vi "Set time.vi"(6 "Defer restart? (true)":bool=TRUE, 8 "error in (no error)":errorcluster, 10 "Time zone":T1 items=["UTC/GMT"=0, "[GMT-1]Azores, Cape Verde"=1, "[GMT-2] Falkland Islands"=2, "[GMT-3] Greenland, East Brazil"=3, "[GMT-4] Central Brazil"=4, "[GMT-5] Eastern United States, Colombia"=5, "[GMT-6] Central United States, Honduras"=6, "[GMT-7] Mountain United States"=7, "[GMT-8] Pacific United States, Yukon"=8, "[GMT-9] Alaska"=9, "[GMT-10] Hawaii, Aleutian Islands"=10, "[GMT-11] Bering Strait"=11, "[GMT+12] New Zealand"=-12, "[GMT+11] Solomon Islands"=-11, "[GMT+10] Eastern Australia"=-10, "[GMT+9] Japan/Korea"=-9, "[GMT+8] Western Australia, Taiwan"=-8, "[GMT+7] Thailand"=-7, "[GMT+6] Central Asia"=-6, "[GMT+5] Pakistan"=-5, "[GMT+4] Gorki, Central Asia, Oman"=-4, "[GMT+3] Turkey, Saudi Arabia"=-3, "[GMT+2] Finland, South Africa"=-2, "[GMT+1] Norway"=-1], 11 "RT Management in":refnum<class "RT Management.lvclass">) -> (0 "error out":errorcluster, 3 "RT Management out":refnum<class "RT Management.lvclass">)   [LabVIEW 2016, in "RT Management.lvlib" / "RT Management.lvclass"]
doc: "Sets the current time and time zone of an RT target. If a reboot is needed, the VI handles the reboot."
uses:
  RT Management.lvclass
  Controls/Time zone.ctl
  RT Management.lvclass/RT Management.ctl
  Get SysCfg Session.vi
  <vilib>/nisyscfg/Close (Hardware).vi
  <resource>/objmgr/niflexriosae.rc
  <resource>/objmgr/nicriosae.rc
  <resource>/objmgr/nisysapi.rc
  <vilib>/nisyscfg/nisyscfg.lvlib
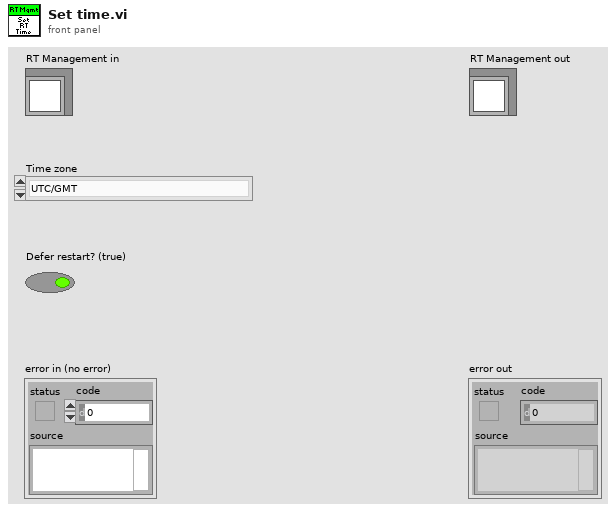
[diagram p1: front panel]
types:
  T1 = typedef "RT Management.lvlib/RT Management.lvclass/Time zone.ctl" = i8
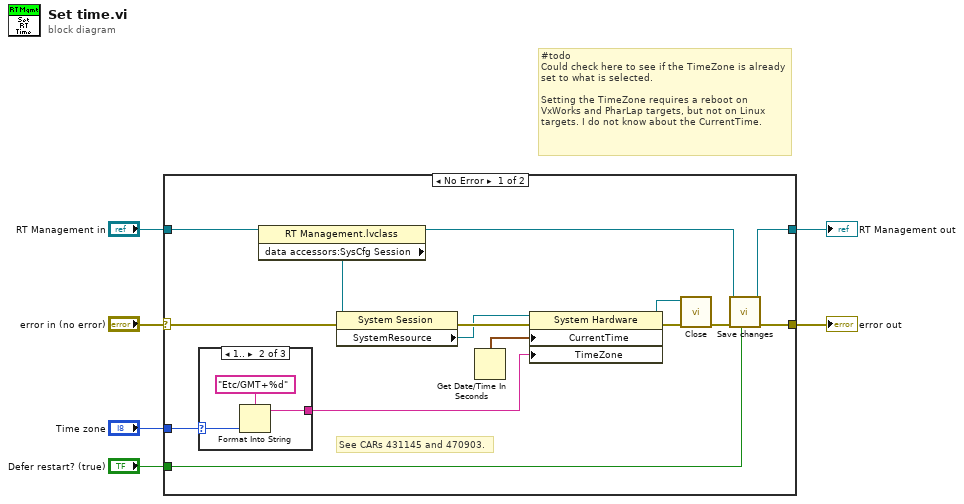
[diagram p0: block diagram]
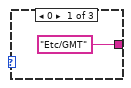
[diagram p2: hidden frame]
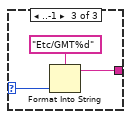
[diagram p3: hidden frame]
diagram:
  # "#todo\nCould check here to see if the TimeZone is already set to what is selected.\n\nSetting the TimeZone requires a reboot on VxWorks and PharLap targets, but not on Linux targets. I do not know about the CurrentTime."
  n1 = case shown="No Error" "error in (no error)" {
    selector: "error in (no error)" -> [w19 w30]
    tunnel: [w20 w30] -> w5
    tunnel: [w18 w29] -> w3
    tunnel: "RT Management in" -> [w21 w29]
    tunnel: "Time zone" -> [w11 _]
    tunnel: "Defer restart? (true)" -> [w17 _]
    frame No Error {
      # "See CARs 431145 and 470903."
      n2 = case shown="1.." w11 {
        selector: w11 -> [_ w23 w26]
        tunnel: ["Etc/GMT" ("format string") w24 w27] -> w9
        frame 0 {
        }
        frame 1.. {
          n3 = Format Into String(format string="Etc/GMT+%d", w23) -> (resulting string=w24:string)  [unwired: 2 in, 1 out]
        }
        frame ..-1 {
          n4 = Format Into String(format string="Etc/GMT%d", w26) -> (resulting string=w27:string)  [unwired: 2 in, 1 out]
        }
      }
      n5 = property class="RT Management.lvclass"(reference=w21) -> (reference out=w13:refnum<class "RT Management.lvclass">, "data accessors:SysCfg Session"=w10:refnum<k21>)  [unwired: 1 in, 1 out]
      n6 = property class="System Session"(reference=w10, error in=w19) -> (error out=w15:errorcluster, "SystemResource"=w12:refnum<k20>)  [unwired: 1 out]
      n7 = Get Date/Time In Seconds() -> (seconds since 1Jan1904=w16:timestamp)
      n8 = property class="System Hardware"(reference=w12, error in=w15, "CurrentTime"=w16, "TimeZone"=w9) -> (reference out=w7:refnum<k20>, error out=w8:errorcluster)
      n9 = call-poly <vilib>:"Close.vi"("error in (no error)"=w8, "Resource in"=w7) -> ("error out"=w14:errorcluster)  [unwired: 9 in]
      n10 = call "Save changes.vi"("Defer restart? (true)"=w17, "error in (no error)"=w14, "RT Management in"=w13) -> ("error out"=w20:errorcluster, "RT Management out"=w18:refnum<class "RT Management.lvclass">)  [unwired: 7 in]
    }
    frame Error {
    }
  }
  "error out" <- w5
  "RT Management out" <- w3
